vi "CH_LM Measurement Fetch Missing Data Count.vi"(0 "Meter Index":i32, 5 "error in (no error)":errorcluster, 7 "Timeout / ms (3000)":i32=3000, 9 "Lock Timeout / ms (1000)":i32=1000) -> (11 "Lock timed out":bool, 14 "Meter Index":i32, 16 "Missing data records":i32, 19 "error out":errorcluster)   [LabVIEW 2012, in "CH_LM.lvlib"]
doc: "This VI queries the number of missing data records due to a measurement data transmission queue full condition."
uses:
  CH_LM.lvlib
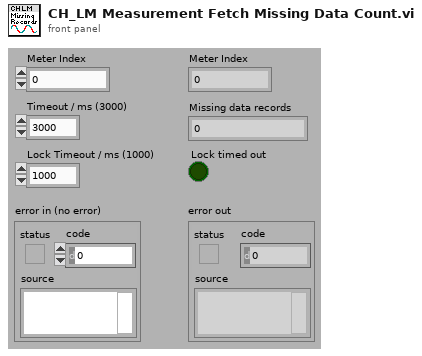
[diagram p1: front panel]
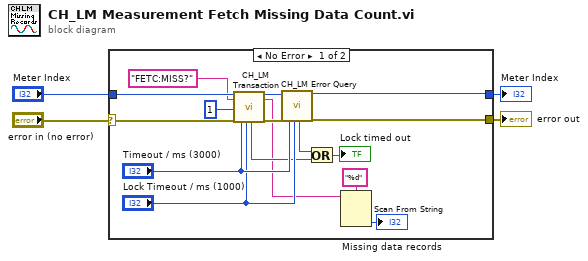
[diagram p0: block diagram]
diagram:
  n1 = case shown="No Error" "error in (no error)" {
    selector: "error in (no error)" -> [w20 w22]
    tunnel: [w13 w22] -> w4
    tunnel: "Meter Index" -> [w19 w21]
    tunnel: [w14 w21] -> w1
    frame No Error {
      n2 = call "CH_LM Transaction.vi"("Meter Index"=w19, "Command String"="FETC:MISS?", "NofStrings (-1:all)"=1, "error in (no error)"=w20, "Timeout / ms (3000)"="Timeout / ms (3000)", "Lock Timeout / ms (1000)"="Lock Timeout / ms (1000)") -> ("Lock timed out"=w9:bool, "Meter Index"=w15:i32, "Response"=w7:string, "error out"=w16:errorcluster)  [unwired: 10 out]
      n3 = call "CH_LM Error Query.vi"("Meter Index"=w15, "error in (no error)"=w16, "Timeout / ms (3000)"="Timeout / ms (3000)", "Lock Timeout / ms (1000)"="Lock Timeout / ms (1000)") -> ("Lock timed out"=w10:bool, "Meter Index"=w14:i32, "error out"=w13:errorcluster)  [unwired: 13 out]
      n4 = Or(x=w10, y=w9) -> (x .or. y?=→"Lock timed out":bool)
      n5 = Scan From String(format string="%d", input string=w7) -> (output 1=→"Missing data records":i32)  [unwired: 2 in, 4 out]
    }
    frame Error {
    }
  }
  "error out" <- w4
  "Meter Index" <- w1
